vi "fronts_ext.vi"(5 "not in old":bool, 7 "in":bool) -> (1 "not in":bool, 2 "fall":bool, 3 "raise":bool)   [LabVIEW 2019, in "Logik.lvlib"]
uses:
  Logik.lvlib
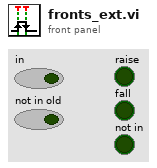
[diagram p1: front panel]
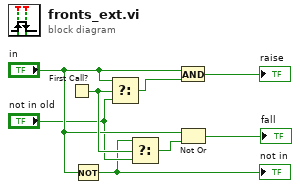
[diagram p0: block diagram]
diagram:
  n1 = First Call?() -> (First Call?: T/F=w6:bool)
  n2 = Not(x="in") -> (.not. x?=w2:bool)
  "not in" <- w2
  n3 = Select(t="in", s=w6, f="not in old") -> (s? t:f=w4:bool)
  n4 = Select(t=w2, s=w6, f="not in old") -> (s? t:f=w1:bool)
  n5 = And(x="in", y=w4) -> (x .and. y?=→"raise":bool)
  n6 = Not Or(1:w1, 2:"in") -> (0:→"fall":bool)
